vi "FindInstruments.vi"(8 "error in (no error)":errorcluster, 11 "KeysightN9020B.lvlib:KeysightN9020B.lvclass":refnum<class "KeysightN9020B.lvclass">) -> (0 "error out":errorcluster, 3 "KeysightN9020B.lvlib:KeysightN9020B.lvclass":refnum<class "KeysightN9020B.lvclass">)   [LabVIEW 2023, in "KeysightN9020B.lvlib" / "KeysightN9020B.lvclass"]
uses:
  KeysightN9020B.lvclass
  KeysightN9020B.lvclass/KeysightN9020B.ctl
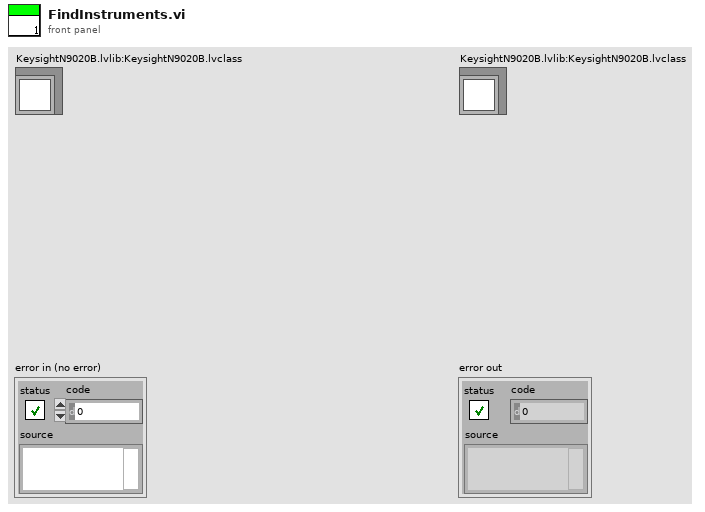
[diagram p1: front panel]
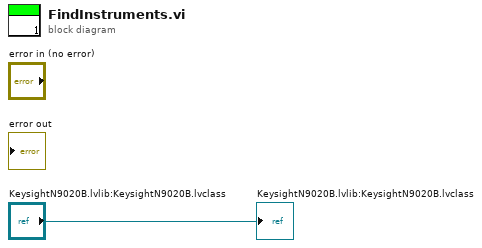
[diagram p0: block diagram]
diagram:
  "KeysightN9020B.lvlib:KeysightN9020B.lvclass" <- "KeysightN9020B.lvlib:KeysightN9020B.lvclass"
